vi "data_ref-waypt_0707-5m decrease.vi"() -> ()   [LabVIEW 2019]
panel:
  out "XY 그래프":cluster{"X":dbl, "Y":dbl}[](graph)
  out "XY 그래프 2":cluster{cluster{"X":dbl, "Y":dbl}[]}[](graph)=[{[{"X"=175630.83485655364, "Y"=530139.7781085183}, {"X"=175630.83363761692, "Y"=530139.7799022729}, {"X"=175630.8322193985, "Y"=530139.7820073679}, {"X"=175630.83101643546, "Y"=530139.7838121755}, {"X"=175630.82981877855, "Y"=530139.7856125266}, {"X"=175630.82842177944, "Y"=530139.7877042423}, {"X"=175630.82724090433, "Y"=530139.789489007}, {"X"=175630.82606533082, "Y"=530139.7912693175}, {"X"=175630.82489329288, "Y"=530139.7930462877}, {"X"=175630.82373186134, "Y"=530139.7948154584}, {"X"=175630.82236758017, "Y"=530139.7968882103}, {"X"=175630.82121237158, "Y"=530139.7986651314}, {"X"=175630.82006245488, "Y"=530139.8004342685}, {"X"=175630.8189231682, "Y"=530139.8022044838}, {"X"=175630.81759077648, "Y"=530139.8042771438}, {"X"=175630.8164762534, "Y"=530139.8060328605}, {"X"=175630.81537231512, "Y"=530139.807774115}, {"X"=175630.81406107475, "Y"=530139.8098100886}, {"X"=175630.81296240148, "Y"=530139.8115335718}, {"X"=175630.81186987998, "Y"=530139.8132403891}, {"X"=175630.81129126588, "Y"=530139.8140866769}, {"X"=175630.81129995524, "Y"=530139.8140289392}, {"X"=175630.8113192468, "Y"=530139.8139611825}, {"X"=175630.81134209206, "Y"=530139.8138978528}, {"X"=175630.81137290265, "Y"=530139.8138322823}, {"X"=175630.8114080731, "Y"=530139.8137422806}, {"X"=175630.8114503338, "Y"=530139.8136544798}, {"X"=175630.811499644, "Y"=530139.8135533386}, {"X"=175630.81156485248, "Y"=530139.8134366126}, {"X"=175630.81162828626, "Y"=530139.8133187837}, {"X"=175630.81169083423, "Y"=530139.8132009557}, {"X"=175630.81174895348, "Y"=530139.8130831408}, {"X"=175630.81180089182, "Y"=530139.8129720043}, {"X"=175630.8118572308, "Y"=530139.8128519747}, {"X"=175630.8119082533, "Y"=530139.8127297421}, {"X"=175630.8119513092, "Y"=530139.8126108615}, {"X"=175630.81199879711, "Y"=530139.812493078}, {"X"=175630.8120444543, "Y"=530139.8123542116}, {"X"=175630.812093661, "Y"=530139.8122175562}, {"X"=175630.812148166, "Y"=530139.812075335}, {"X"=175630.81212503387, "Y"=530139.8120409976}, {"X"=175630.8118207068, "Y"=530139.8121728477}, {"X"=175630.81046722573, "Y"=530139.8127838852}, {"X"=175630.8073735051, "Y"=530139.8141202934}, {"X"=175630.8020442867, "Y"=530139.8164521005}, {"X"=175630.79403494642, "Y"=530139.8200969121}, {"X"=175630.7830349662, "Y"=530139.8251921466}, {"X"=175630.7689638062, "Y"=530139.8317591269}, {"X"=175630.75217447654, "Y"=530139.8396536494}, {"X"=175630.73268868006, "Y"=530139.848725824}, {"X"=175630.71068133102, "Y"=530139.8588108785}, {"X"=175630.68679259712, "Y"=530139.8698214887}, {"X"=175630.66210180896, "Y"=530139.8816024584}, {"X"=175630.6370555141, "Y"=530139.893582021}, {"X"=175630.61279362146, "Y"=530139.9051175728}, {"X"=175630.59006113734, "Y"=530139.9162280303}, {"X"=175630.5687154615, "Y"=530139.9263089383}, {"X"=175630.5492750472, "Y"=530139.9354508994}, {"X"=175630.5310082024, "Y"=530139.9442531541}, {"X"=175630.51281634127, "Y"=530139.9526456536}, {"X"=175630.49481900368, "Y"=530139.9609177203}, {"X"=175630.476705017, "Y"=530139.9698915594}, {"X"=175630.45770170673, "Y"=530139.9791731995}, {"X"=175630.43736853378, "Y"=530139.9886607106}, {"X"=175630.4162177506, "Y"=530139.9987477091}, {"X"=175630.39433380004, "Y"=530140.009230843}, {"X"=175630.37174333088, "Y"=530140.0198314639}, {"X"=175630.3489954596, "Y"=530140.0308287616}, {"X"=175630.32593544153, "Y"=530140.0420100953}, {"X"=175630.30204959612, "Y"=530140.0534036001}, {"X"=175630.27753325136, "Y"=530140.0651640864}, {"X"=175630.25178450788, "Y"=530140.0774431387}, {"X"=175630.2248458256, "Y"=530140.0905236471}, {"X"=175630.1970098615, "Y"=530140.1042205227}, {"X"=175630.16815773962, "Y"=530140.1178659785}, {"X"=175630.13922927048, "Y"=530140.1314517233}, {"X"=175630.110838787, "Y"=530140.1448405647}, {"X"=175630.08384356435, "Y"=530140.1579734028}, {"X"=175630.05785717693, "Y"=530140.1707725613}, {"X"=175630.03256878696, "Y"=530140.1829625951}, {"X"=175630.0079059243, "Y"=530140.1945992041}, {"X"=175629.9837209854, "Y"=530140.2060956879}, {"X"=175629.95993842997, "Y"=530140.21767313}, {"X"=175629.9358164363, "Y"=530140.2294935079}, {"X"=175629.9112739501, "Y"=530140.2414016835}, {"X"=175629.88643384873, "Y"=530140.2533140553}, {"X"=175629.86093668928, "Y"=530140.2655990346}, {"X"=175629.83472129318, "Y"=530140.2782357128}, {"X"=175629.80741847897, "Y"=530140.2912917578}, {"X"=175629.77915645548, "Y"=530140.3049909872}, {"X"=175629.74996227038, "Y"=530140.3191923694}, {"X"=175629.71972566724, "Y"=530140.3337519446}, {"X"=175629.6890004814, "Y"=530140.348440578}, {"X"=175629.65781094748, "Y"=530140.3633669652}, {"X"=175629.62668956464, "Y"=530140.3785783864}, {"X"=175629.59531305832, "Y"=530140.3937838941}, {"X"=175629.56387973213, "Y"=530140.4089451723}, {"X"=175629.53244943306, "Y"=530140.4242340742}, {"X"=175629.50119149982, "Y"=530140.4393970617}, {"X"=175629.47013264612, "Y"=530140.4544839975}, {"X"=175629.43956165554, "Y"=530140.4694995914}, {"X"=175629.4093964925, "Y"=530140.4845606147}, {"X"=175629.37936374222, "Y"=530140.4994658756}, {"X"=175629.34936506223, "Y"=530140.5142067751}, {"X"=175629.31939175382, "Y"=530140.5291440466}, {"X"=175629.28902616276, "Y"=530140.5444276285}, {"X"=175629.257973798, "Y"=530140.5596133235}, {"X"=175629.22634253916, "Y"=530140.5749405479}, {"X"=175629.1943114367, "Y"=530140.590755057}, {"X"=175629.16182733022, "Y"=530140.6070525653}, {"X"=175629.12874200233, "Y"=530140.6234295141}, {"X"=175629.0950809071, "Y"=530140.6398059251}, {"X"=175629.06108796183, "Y"=530140.6562920678}, {"X"=175629.02683541513, "Y"=530140.6730608717}, {"X"=175628.99260259036, "Y"=530140.6899095266}, {"X"=175628.9582281093, "Y"=530140.7067830133}, {"X"=175628.92393588362, "Y"=530140.7233088734}, {"X"=175628.890190515, "Y"=530140.7396433549}, {"X"=175628.8568507918, "Y"=530140.7559600053}, {"X"=175628.82383025042, "Y"=530140.7723789434}, {"X"=175628.7913323974, "Y"=530140.7885188934}, {"X"=175628.75929107613, "Y"=530140.8044743862}, {"X"=175628.7275717504, "Y"=530140.8205843191}, {"X"=175628.69560178922, "Y"=530140.8367094123}, {"X"=175628.66345296457, "Y"=530140.8528583344}, {"X"=175628.6314678988, "Y"=530140.8692720344}, {"X"=175628.59933777034, "Y"=530140.885451979}, {"X"=175628.56731660504, "Y"=530140.9016360445}, {"X"=175628.535215808, "Y"=530140.9178514162}, {"X"=175628.50308388958, "Y"=530140.9343288087}, {"X"=175628.47046066754, "Y"=530140.950914177}, {"X"=175628.4373826674, "Y"=530140.9676762302}, {"X"=175628.40404248016, "Y"=530140.9844423775}, {"X"=175628.3706110085, "Y"=530141.0011910326}, {"X"=175628.3373002241, "Y"=530141.0180148073}, {"X"=175628.30416979874, "Y"=530141.0347215208}, {"X"=175628.2712462234, "Y"=530141.0518893327}, {"X"=175628.23819644627, "Y"=530141.0686102388}, {"X"=175628.20533112012, "Y"=530141.0854016393}, {"X"=175628.17244429275, "Y"=530141.1018057605}, {"X"=175628.14000352132, "Y"=530141.118685823}, {"X"=175628.10800383775, "Y"=530141.1358576022}, {"X"=175628.0761047121, "Y"=530141.1528848062}, {"X"=175628.04411354283, "Y"=530141.1696348138}, {"X"=175628.01207426272, "Y"=530141.1868966075}, {"X"=175627.98016569787, "Y"=530141.204331158}, {"X"=175627.94803915342, "Y"=530141.2214367153}, {"X"=175627.91579747843, "Y"=530141.2382462752}, {"X"=175627.8835852169, "Y"=530141.2551179036}, {"X"=175627.85138831387, "Y"=530141.2723956952}, {"X"=175627.81898504467, "Y"=530141.2896829674}, {"X"=175627.78638904754, "Y"=530141.3070973236}, {"X"=175627.75382836853, "Y"=530141.3244738434}, {"X"=175627.7215711273, "Y"=530141.3420203964}, {"X"=175627.68934733944, "Y"=530141.3591917201}, {"X"=175627.65695085836, "Y"=530141.3763757573}, {"X"=175627.62447569822, "Y"=530141.3936132942}, {"X"=175627.59172904206, "Y"=530141.4113055577}, {"X"=175627.558773741, "Y"=530141.4291371601}, {"X"=175627.52549546957, "Y"=530141.4467821376}, {"X"=175627.49262329255, "Y"=530141.4648687661}, {"X"=175627.4603627449, "Y"=530141.4837116452}, {"X"=175627.42847909738, "Y"=530141.5030084677}, {"X"=175627.3962783145, "Y"=530141.521690244}, {"X"=175627.36414483137, "Y"=530141.5400610629}, {"X"=175627.33237347484, "Y"=530141.558376444}, {"X"=175627.30117397054, "Y"=530141.5768677343}, {"X"=175627.27039708497, "Y"=530141.5947851066}, {"X"=175627.23997753716, "Y"=530141.6125227505}, {"X"=175627.20974048215, "Y"=530141.6302676313}, {"X"=175627.17896778567, "Y"=530141.6477987617}, {"X"=175627.14769317146, "Y"=530141.6657453316}, {"X"=175627.11586873207, "Y"=530141.684081955}, {"X"=175627.08343074302, "Y"=530141.702523583}, {"X"=175627.05065172852, "Y"=530141.7215744087}, {"X"=175627.01737871178, "Y"=530141.7404135825}, {"X"=175626.9838281253, "Y"=530141.7594477901}, {"X"=175626.9505958465, "Y"=530141.7788906071}, {"X"=175626.91748777666, "Y"=530141.7980988838}, {"X"=175626.88475178962, "Y"=530141.8170208395}, {"X"=175626.85316989815, "Y"=530141.8365176701}, {"X"=175626.82268731782, "Y"=530141.8566372552}, {"X"=175626.79267880594, "Y"=530141.8759041985}, {"X"=175626.76302988536, "Y"=530141.8951567747}, {"X"=175626.7335929421, "Y"=530141.9145030702}, {"X"=175626.70371870397, "Y"=530141.9339471988}, {"X"=175626.6736656086, "Y"=530141.9537203669}, {"X"=175626.64270664734, "Y"=530141.9732919617}, {"X"=175626.61134064768, "Y"=530141.9933142383}, {"X"=175626.57972040272, "Y"=530142.0142395666}, {"X"=175626.54731397808, "Y"=530142.0346966096}, {"X"=175626.5146245485, "Y"=530142.0553065287}, {"X"=175626.48195363258, "Y"=530142.0758864263}, {"X"=175626.449574957, "Y"=530142.096442166}, {"X"=175626.41787400912, "Y"=530142.1170303357}, {"X"=175626.38627436184, "Y"=530142.1371209942}, {"X"=175626.354876592, "Y"=530142.1568792148}, {"X"=175626.32392118085, "Y"=530142.1770612239}, {"X"=175626.29313971248, "Y"=530142.1964436265}, {"X"=175626.26268644322, "Y"=530142.2159815638}]}, ...(2 in all)]
  in  "인덱스":i32=200
  in  "정지":bool
  out "크기":i32=10727
  out "XY 그래프 3":cluster{"X":dbl, "Y":dbl}[](graph)
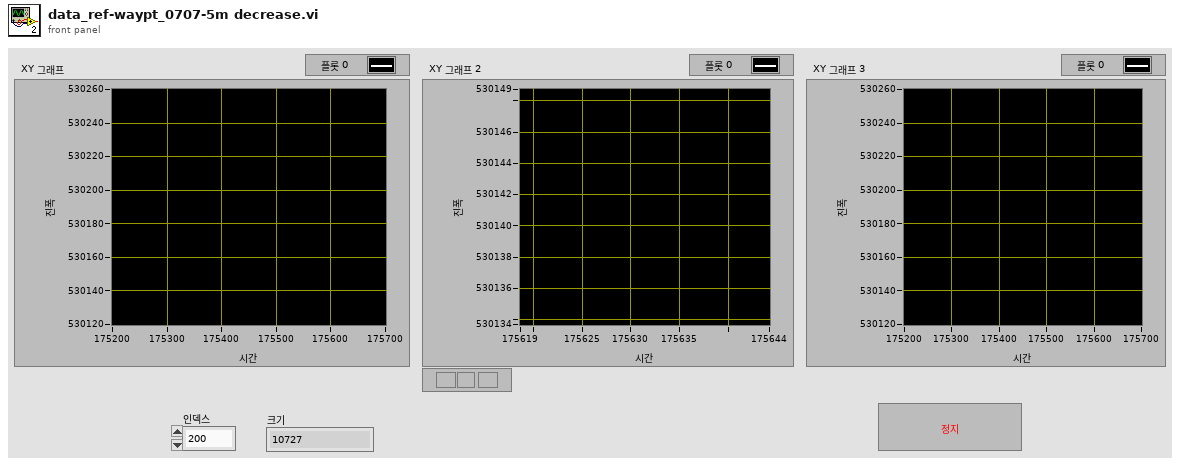
[diagram p1: front panel]
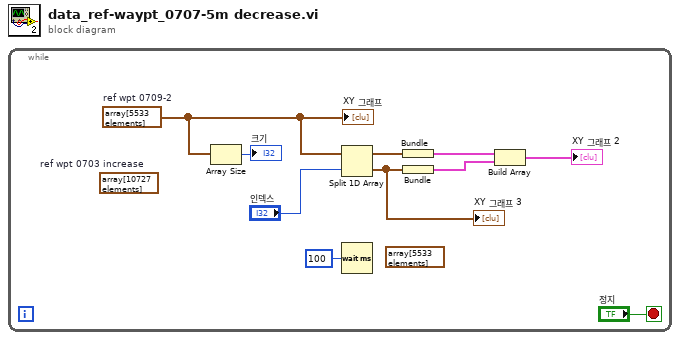
[diagram p0: block diagram]
diagram:
  n1 = while {
    stop <- "정지" stop-if-true
    (unwired) cluster{"X":dbl, "Y":dbl}[] array[5533 elements] ("XY 그래프 4")
    w1 = cluster{dbl, dbl}[] array[5533 elements]  # ref wpt 0709-2
    (unwired) cluster{"X":dbl, "Y":dbl}[] array[10727 elements]  # ref wpt 0703 increase
    n2 = Array Size(array=w1) -> (size(s)=→"크기":i32)
    n3 = Split 1D Array(array=w1, index="인덱스") -> (first subarray=w9:cluster{dbl, dbl}[], second subarray=w2:cluster{dbl, dbl}[])
    "XY 그래프 3" <- w2
    n4 = Wait (ms)(milliseconds to wait=u32 100 ("대기 시간 (ms)")) -> ()  [unwired: 1 out]
    n5 = Bundle(w9) -> (w8:cluster{cluster{dbl, dbl}[]})  [unwired: 1 in]
    n6 = Bundle(w2) -> (w3:cluster{cluster{dbl, dbl}[]})  [unwired: 1 in]
    n7 = Build Array(w8, w3) -> (→"XY 그래프 2":cluster{cluster{dbl, dbl}[]}[])
    "XY 그래프" <- w1
  }
